vi "Read DIO Channel Setting.vi"(8 "error in (no error)":errorcluster, 11 "DIO Channel configuration in":refnum<class "Digital IO Channel configuration.lvclass">) -> (0 "error out":errorcluster, 2 "DIO Channel Setting":T1, 3 "DIO Channel configuration out":refnum<class "Digital IO Channel configuration.lvclass">)   [LabVIEW 2025, in "Digital IO.lvlib" / "Digital IO Channel configuration.lvclass"]
uses:
  Digital IO Channel configuration.lvclass
  DIO Channel Setting.ctl
  Digital IO Channel configuration.lvclass/Digital IO Channel configuration.ctl
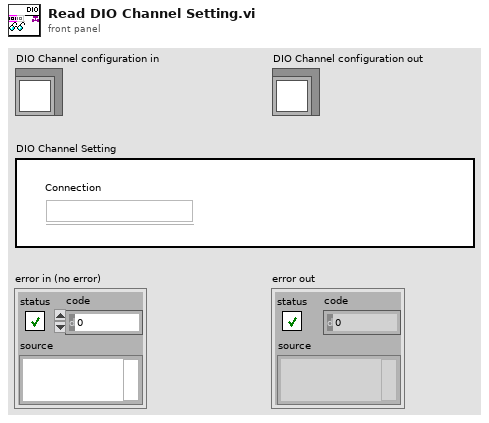
[diagram p1: front panel]
types:
  T1 = typedef "Digital IO.lvlib/Digital IO Channel configuration.lvclass/DIO Channel Setting.ctl" = cluster{"Connection":string}
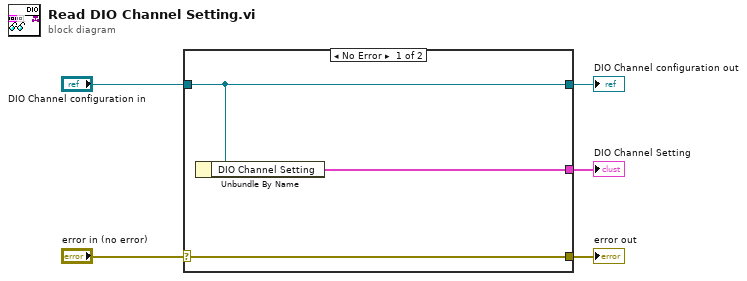
[diagram p0: block diagram]
diagram:
  n1 = case shown="No Error" "error in (no error)" {
    selector: "error in (no error)" -> [w8 w9]
    tunnel: [w8 w9] -> w4
    tunnel: [w7 w10] -> w2
    tunnel: "DIO Channel configuration in" -> [w7 w10]
    tunnel: [w6 _] -> w1
    frame No Error {
      n2 = Unbundle By Name(w7) -> ("DIO Channel Setting"=w6:T1)
    }
    frame Error {
    }
  }
  "error out" <- w4
  "DIO Channel configuration out" <- w2
  "DIO Channel Setting" <- w1
